vi "Create Default Attributes.vi"(5 "Unique ID":string, 7 "Process Executive Ref":refnum<data-value>, 11 "Start High Pressure Wash in":refnum<class "Start High Pressure Wash.lvclass">) -> (3 "Start High Pressure Wash out":refnum<class "Start High Pressure Wash.lvclass">)   [LabVIEW 2019, in "Start High Pressure Wash.lvclass"]
uses:
  <vilib>/gpm_packages/@cs/Car-wash/Source/Process Steps/Start High Pressure Wash/Start High Pressure Wash.lvclass
  <vilib>/gpm_packages/@cs/test-executive/Source/Test Executive/ITestExecutive/ITest Executive.lvclass
  9611c926-e529-4d62-8d59-916b17f8f3d4.vi
  <vilib>/Utility/error.llb/Error Cluster From Error Code.vi
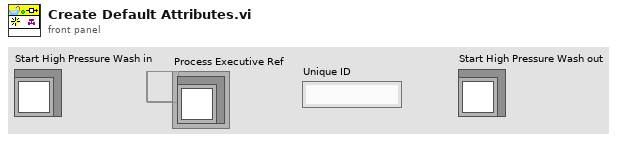
[diagram p1: front panel]
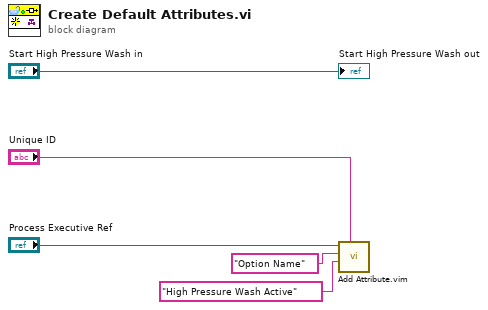
[diagram p0: block diagram]
diagram:
  n1 = call "Add Attribute.vim"("ID"="Unique ID", "Attribute"="High Pressure Wash Active" ("Item Name"), "Attribute Name"="Option Name" ("Item Name"), "Test Executive Ref"="Process Executive Ref") -> ()  [unwired: 4 in, 4 out]
  "Start High Pressure Wash out" <- "Start High Pressure Wash in"
